vi "g_GPCounters.vi"() -> ()   [LabVIEW 2014]
panel:
  out "Counter 3":dbl
  out "Counter 2":dbl
  out "Counter 1":dbl
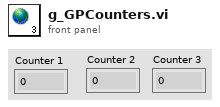
[diagram p1: front panel]
diagram:
